vi "FA_ConvertFromConfigItemData.vi"(8 "Error In":errorcluster, 11 "Items":T1) -> (0 "Error Out":errorcluster, 3 "XML String":string)   [LabVIEW 2014, in "FA_NativeTypes.lvlib"]
doc: "Converts from the Items typedef to an XML string"
uses:
  FA_NativeTypes.lvlib
  FA_ConfigItem.ctl
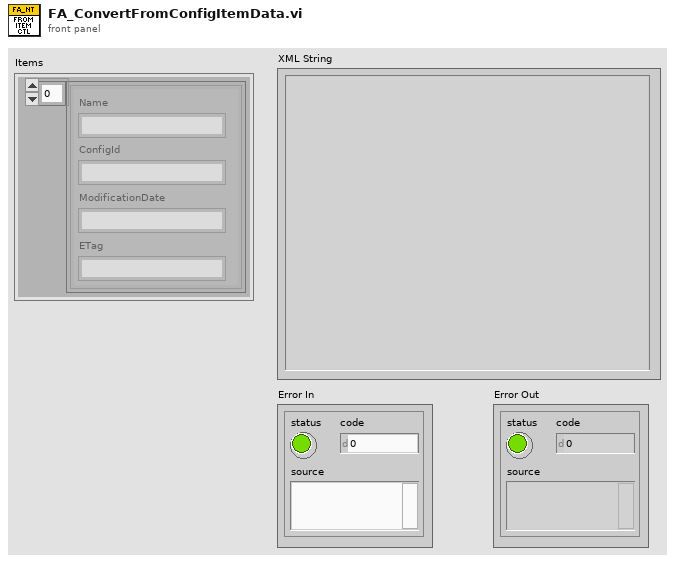
[diagram p1: front panel]
types:
  T1 = typedef "FA_NativeTypes.lvlib/FA_ConfigItem.ctl" = cluster{"Item":cluster{"Name":string, "ConfigId":string, "ModificationDate":string, "ETag":string}[]}
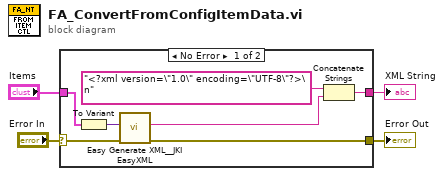
[diagram p0: block diagram]
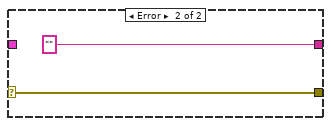
[diagram p2: hidden frame]
diagram:
  n1 = case shown="No Error" "Error In" {
    selector: "Error In" -> [w11 w13]
    tunnel: [w8 w13] -> w3
    tunnel: "Items" -> [w9 _]
    tunnel: [w5 "" ("XML String")] -> w2
    frame No Error {
      n2 = To Variant(anything=w9) -> (Variant=w10:variant)
      n3 = call <vilib>:"Easy Generate XML__JKI EasyXML.vi"("error in (no error)"=w11, "LabVIEW Data"=w10) -> ("error out"=w8:errorcluster, "XML String"=w7:string)  [unwired: 8 in]
      n4 = Concatenate Strings("<?xml version=\"1.0\" encoding=\"UTF-8\"?>\n" ("string"), w7) -> (w5:string)
    }
    frame Error {
    }
  }
  "Error Out" <- w3
  "XML String" <- w2
